vi "Read Async Call Method.vi"(8 "error in (no error)":errorcluster, 11 "Async Message Msg in":refnum<class "Async Message.lvclass">) -> (0 "error out":errorcluster, 2 "Async Method":T1, 3 "Async Message Msg out":refnum<class "Async Message.lvclass">)   [LabVIEW 2021, in "Async Methods Actor.lvlib" / "Async Message.lvclass"]
uses:
  Async Message.lvclass
  Async Methods Actor/Async Call Method.ctl
  Async Message.lvclass/Async Message.ctl
  Async Methods Actor/Async Methods Actor.lvclass
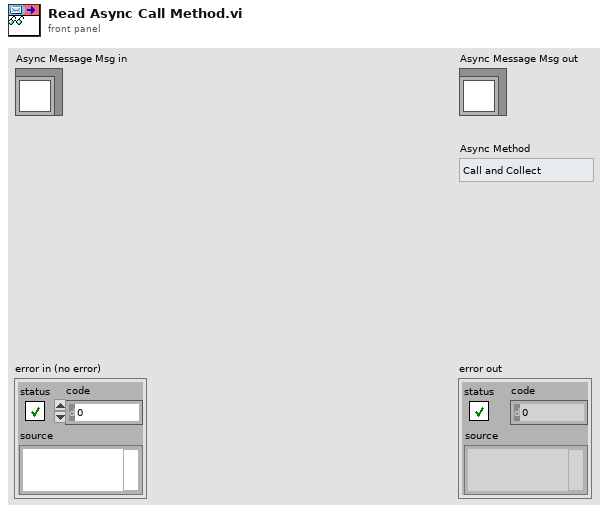
[diagram p1: front panel]
types:
  T1 = typedef "Async Methods Actor.lvlib/Async Methods Actor.lvclass/Async Call Method.ctl" = enum16{"Call and Collect", "Call and Forget"}
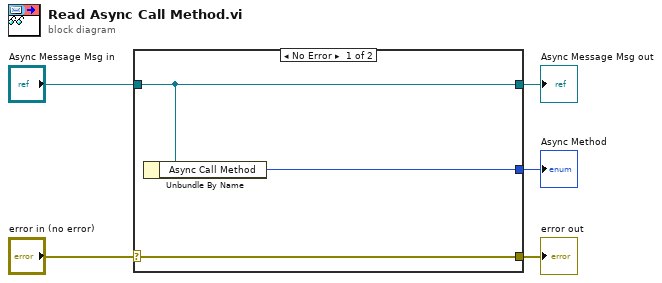
[diagram p0: block diagram]
diagram:
  n1 = case shown="No Error" "error in (no error)" {
    selector: "error in (no error)" -> [w8 w9]
    tunnel: [w8 w9] -> w4
    tunnel: [w7 w10] -> w2
    tunnel: "Async Message Msg in" -> [w7 w10]
    tunnel: [w6 _] -> w1
    frame No Error {
      n2 = Unbundle By Name(w7) -> ("Async Call Method"=w6:T1)
    }
    frame Error {
    }
  }
  "error out" <- w4
  "Async Message Msg out" <- w2
  "Async Method" <- w1
